vi "Plot Helper.vi"   [LabVIEW 2017, in "3D Contour Datatype.lvclass"]
doc: "Graphs a plot with contour lines. Multiple references to this VI generate multiple plots for the same graph."
uses:
  <vilib>/Math Plots/3D Math Plots/3D Contour/3D Contour Datatype/3D Contour Datatype.lvclass
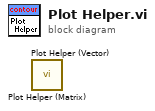
[diagram p0: block diagram]
diagram:
  n1 = call <vilib>:"Plot Helper (Matrix).vi"() -> ()  [unwired: 10 in, 2 out]
  n2 = call <vilib>:"Plot Helper (Vector).vi"() -> ()  [unwired: 10 in, 2 out]
